vi "AdvancedConfig.vi"(8 "Error In":errorcluster, 11 "Config In":T1={"DAQ"={"Data"={"Live"={"t0"=timestamp(0 s since 1904-01-01), "dt"=1.0, "Y"=[]}, "Accumulated"={"t0"=timestamp(0 s since 1904-01-01), "dt"=1.0, "Y"=[]}, "Averaged"={"t0"=timestamp(0 s since 1904-01-01), "dt"=1.0, "Y"=[]}, "data array"=[], "live time array"=[], "Live (decimated)"={"t0"=timestamp(0 s since 1904-01-01), "dt"=1.0, "Y"=[]}}, "Config"={"Input Config"=0, "Card"=enum."USB-6211", "100% Reflectance Standard (V)"=0.0, "Input Channel"="Dev1/ai0", "Average number of points"=0.0, "Trigger Level (V)"=0.0, "Rate (Hz)"=0, "End Time (s)"=0.0}, "Indicators"={"Final number of points"=0.0, "Number of samples"=0.0, "dt"=0.0, "Shots"=0, "Shot counter"=0, "Test counter"=0, "Background level (V)"=0.0, "DAQ task"="", "timestamp of data"=timestamp(0 s since 1904-01-01), "Test Type"=enum."A-Test"}}, "Shutter"={"Open command string"="", "VISA"={"Timeout (ms)"=0, "Resource Name"="", "Baud Rate"=0, "Data Bits"=0, "Parity"=0, "Stop Bits"=0, "Flow Control"=0}}, "Monochromator"={"Type"=enum."Oriel", "Wavelength (nm)"=0.0, "Grating, gr/mm"=enum."2400", "Grating mode"=enum."Unknown", "Spectrum mode"={"Spectrum mode?"=FALSE, "Start wavelength (nm)"=0.0, "End wavelength (nm)"=0.0, "Wavelength step (nm)"=0.0, "Wavelength array"=[], "array index"=0}, "PTI"={"Delay before read (ms)"=0, "Mono 1"={"Timeout (ms)"=0, "Resource Name"="", "Baud Rate"=0, "Data Bits"=0, "Parity"=0, "Stop Bits"=0, "Flow Control"=0}, "Mono 2"={"Timeout (ms)"=0, "Resource Name"="", "Baud Rate"=0, "Data Bits"=0, "Parity"=0, "Stop Bits"=0, "Flow Control"=0}, "Two PTI Monochromators?"=FALSE}, "Oriel (custom)"={"reference"=refnum}, "Force wavelength confirmation (PTI)?"=FALSE}, "Test"={"Config"={"Amplification Factor"=0.0, "100% Reflectance Standard"=0.0, "Calculation Method"=enum."Reflectance", "Option to discard new data?"=FALSE, "Mode"=enum."Spectrum", "Number of Averages"=0, "B Test?"=FALSE}, "Indicators"={"DAQ Background Level (V)"=0.0, "A-Test Counter"=0, "B-Test Counter"=0, "Type"=enum."A-Test", "Scope Background Level (Amps)"=2.0, "TAS only?"=FALSE}}, "Scope"={"Config"={"VISA Resource"="", "Model"=enum."DPO 3012", "Timebase"=0.0, "Timeout (ms)"=0, "TAS"={"Vertical Range (V)"=0.0, "Vertical Offset (0.0 divs)"=0.0, "Bandwidth"=0, "Probe Attenuation (10.0)"=0.0, "Vertical Coupling"=0, "Impedance"=0, "Multiplication factor"=0.0, "Channel"=enum."Channel 1"}, "TPC"={"Vertical Range (V)"=0.0, "Vertical Offset (0.0 divs)"=0.0, "Bandwidth"=0, "Probe Attenuation (10.0)"=0.0, "Vertical Coupling"=0, "Impedance"=0, "Multiplication factor"=0.0, "Channel"=enum."Channel 1"}, "Trigger"={"Mode"=enum."Laser (TAS)", "Source "=enum."Channel 1", "PIA"={"Test LEDs"=FALSE, "LED line"="", "LED off (s)"=0.0, "LED on (s)"=0.0}, "Threshold (V)"=0.0}}, "Indicators"={"Setup"={"Final number of points"=0.0, "Pretrigger points"=0.0, "Number of readouts"=0, "Model"={"Acquisition Type"=0, "Record length (points)"=0, "Averages on scope"=0, "Average number of points"=0.0}}, "Timestamp of Data"=timestamp(0 s since 1904-01-01)}, "Data"={"TPC"={"Live data"={"t0"=timestamp(0 s since 1904-01-01), "dt"=1.0, "Y"=[]}, "Averaged data"={"t0"=timestamp(0 s since 1904-01-01), "dt"=1.0, "Y"=[]}, "Accumulated data"={"t0"=timestamp(0 s since 1904-01-01), "dt"=1.0, "Y"=[]}, "Final data"={"t0"=timestamp(0 s since 1904-01-01), "dt"=1.0, "Y"=[]}}, "TAS"={"Live data"={"t0"=timestamp(0 s since 1904-01-01), "dt"=1.0, "Y"=[]}, "Averaged data"={"t0"=timestamp(0 s since 1904-01-01), "dt"=1.0, "Y"=[]}, "Accumulated data"={"t0"=timestamp(0 s since 1904-01-01), "dt"=1.0, "Y"=[]}, "Final data"={"t0"=timestamp(0 s since 1904-01-01), "dt"=1.0, "Y"=[]}}, "Time arrays"={"Time array (decimated)"=[], "waveform"={"t0"=timestamp(0 s since 1904-01-01), "dt"=1.0, "Y"=[]}}}, "Test"={"Config"={"Amplification Factor"=2.0, "100% Reflectance Standard"=2.0, "Calculation Method"=enum."Reflectance", "Option to discard new data?"=FALSE, "Mode"=enum."Spectrum", "Number of Averages"=0, "B Test?"=FALSE}, "Indicators"={"DAQ Background Level (V)"=2.0, "A-Test Counter"=2, "B-Test Counter"=2, "Type"=enum."A-Test", "Scope Background Level (Amps)"=2.0, "TAS only?"=FALSE}}}, "Colour wheel"={"Reference"=0, "Colour Wheel Wavelengths"=[], "Waveform Index"=0, "COM Port"="", "Enabled?"=FALSE}, "File IO"={"Output Folder"=path "", "Error file"=path "", "Config file"=path "", "File prefix"="", "Waveform read"={"t0"=timestamp(0 s since 1904-01-01), "dt"=1.0, "Y"=[]}}} {"Scope"."Test"."Config"."Number of Averages" min=0; "Scope"."Indicators"."Setup"."Model"."Record length (points)" items=["1000"=1, "10,000"=10, "100,000"=100, "1,000,000"=1000, "5,000,000"=5000, "10,000,000"=10000]; "Scope"."Indicators"."Setup"."Model"."Acquisition Type" items=["Sample", "Peak Detect", "Hi Res", "Envelope", "Average"]; "Scope"."Config"."Trigger"."Threshold (V)" format="%#_3f"; "Scope"."Config"."TPC"."Impedance" items=["1M", "75", "50"]; "Scope"."Config"."TPC"."Vertical Coupling" items=["AC", "DC", "Ground"]; "Scope"."Config"."TPC"."Bandwidth" items=["FULL", "250 MHz", "150 MHz", "20 MHz"]; "Scope"."Config"."TAS"."Impedance" items=["1M", "75", "50"]; "Scope"."Config"."TAS"."Vertical Coupling" items=["AC", "DC", "Ground"]; "Scope"."Config"."TAS"."Bandwidth" items=["FULL", "250 MHz", "150 MHz", "20 MHz"]; "Scope"."Config"."Timebase" format="%^#_3e"; "Test"."Config"."Number of Averages" min=0; "Monochromator"."PTI"."Mono 2"."Flow Control" items=["1.0"=10, "1.5"=15, "2.0"=20]; "Monochromator"."PTI"."Mono 2"."Stop Bits" items=["None", "Odd", "Even", "Mark", "Space"]; "Monochromator"."PTI"."Mono 2"."Parity" items=["None", "Odd", "Even", "Mark", "Space"]; "Monochromator"."PTI"."Mono 1"."Flow Control" items=["1.0"=10, "1.5"=15, "2.0"=20]; "Monochromator"."PTI"."Mono 1"."Stop Bits" items=["None", "Odd", "Even", "Mark", "Space"]; "Monochromator"."PTI"."Mono 1"."Parity" items=["None", "Odd", "Even", "Mark", "Space"]; "Shutter"."VISA"."Flow Control" items=["None"=0, "XON/XOFF"=1, "RTS/CTS"=2, "DTR/DSR"=4]; "Shutter"."VISA"."Stop Bits" items=["1.0"=10, "1.5"=15, "2.0"=20]; "Shutter"."VISA"."Parity" items=["None", "Odd", "Even", "Mark", "Space"]; "DAQ"."Config"."Input Config" items=["default"=-1, "RSE"=10083, "NRSE"=10078, "Differential"=10106, "Pseudodifferential"=12529]}) -> (0 "Error Out":errorcluster)   [LabVIEW 2017, in "UI.lvlib"]
uses:
  UI.lvlib
  Controls/Move shutter button.ctl
  System Control/CTLs/Params.ctl
  DAQ/Controls/Params.ctl
  DAQ/Controls/DAQ Config.ctl
  DAQ/Controls/DAQ Indicators.ctl
  System Control/CTLs/Test Type.ctl
  Shutter Module/Controls/Params.ctl
  Monochromator/Controls/VISA parameters.ctl
  Monochromator/Controls/Params.ctl
  Monochromator/Controls/Type.ctl
  Monochromator/Controls/GratingValues.ctl
  Monochromator/Controls/Grating.ctl
  Monochromator/PTI/Controls/Params.ctl
  Monochromator/Custom Oriel drivers/Controls/Params.ctl
  C:/Optical Software Code V1.6.1.1/Optical Software Code/Modules/Monochromator/Cornerstone.dll
  Monochromator/Cornerstone.dll
  System Control/CTLs/Test params.ctl
  System Control/CTLs/Test Controls.ctl
  System Control/CTLs/Test indicators.ctl
  Scope/Controls/Params.ctl
  Scope/Controls/Models.ctl
  Scope/Controls/TPC.ctl
  Scope/Controls/Channels.ctl
  Trigger/Controls/Params.ctl
  Trigger/Controls/Mode.ctl
  Trigger/Controls/Trigger channels.ctl
  Scope/Controls/Acquisition type.ctl
  Scope/Controls/Record length.ctl
  Scope/Controls/Data.ctl
  Scope/Controls/Channel data.ctl
  Colour Wheel/Controls/Params.ctl
  File IO/Controls/Params.ctl
  Controls/Config Command [enum].ctl
  File IO/Controls/Config Cluster.ctl
  Shutter Module/Shutter.lvlib
  File IO/File IO.lvlib
  <vilib>/Utility/config.llb/NI_LVConfig.lvlib
  Colour Wheel/Colour Wheel.lvlib
  System Control/Main controller.lvlib
  Trigger/Trigger.lvlib
  Scope/Scope.lvlib
  Monochromator/Custom Oriel drivers/Oriel (custom drivers).lvlib
  Serial comms/Serial comms.lvlib
  Monochromator/PTI/PTI.lvlib
  Monochromator/Monochromator.lvlib
  DAQ/DAQ.lvlib
panel:
  out "Current Config:":path
  in  "Load Config Button":bool
  in  "Save Config Button":bool
  in  "Exit Button":bool
  in  "Tab Control":T30(tab)=enum."Colour Wheel"
  in  "Error Log File":path
  out "Pretrigger points":dbl
  out "Final number of points":dbl
  in  "Scope.Config":T31 {"Trigger"."Threshold (V)" format="%#_3f"; "TPC"."Impedance" items=["1M", "75", "50"]; "TPC"."Vertical Coupling" items=["AC", "DC", "Ground"]; "TPC"."Bandwidth" items=["FULL", "250 MHz", "150 MHz", "20 MHz"]; "TAS"."Impedance" items=["1M", "75", "50"]; "TAS"."Vertical Coupling" items=["AC", "DC", "Ground"]; "TAS"."Bandwidth" items=["FULL", "250 MHz", "150 MHz", "20 MHz"]}
  in  "Scope Model Settings":T32 {"Record length (points)" items=["1000"=1, "10,000"=10, "100,000"=100, "1,000,000"=1000, "5,000,000"=5000, "10,000,000"=10000]; "Acquisition Type" items=["Sample", "Peak Detect", "Hi Res", "Envelope", "Average"]}
  in  "DAQ Controls":T3={"Input Config"=10106, "Card"=enum."USB-6251", "100% Reflectance Standard (V)"=1.0, "Input Channel"="Dev1/ai0", "Average number of points"=10.0, "Trigger Level (V)"=0.2, "Rate (Hz)"=1250000, "End Time (s)"=10.0} {"Input Config" items=["default"=-1, "RSE"=10083, "NRSE"=10078, "Differential"=10106, "Pseudodifferential"=12529]}
  out "DAQ Indicators":T4={"Final number of points"=100.0, "Number of samples"=10000.0, "dt"=5e-06, "Shots"=10, "Shot counter"=10, "Test counter"=10, "Background level (V)"=0.0, "DAQ task"="", "timestamp of data"=timestamp(0 s since 1904-01-01), "Test Type"=enum."A-Test"}
  in  "Desired Wavelength:":dbl min=0.0 max=1600.0 step=1.0
  in  "Move Monochromator Button":bool
  in  "Monochromator Type":T9=enum."PTI"
  in  "Wavelength (nm)":dbl
  in  "Grating, gr/mm":T10
  in  "Monochromator Grating mode":T11=enum."IR"
  in  "PTI":T12={"Delay before read (ms)"=50, "Mono 1"={"Timeout (ms)"=1000, "Resource Name"="COM1", "Baud Rate"=9600, "Data Bits"=8, "Parity"=0, "Stop Bits"=10, "Flow Control"=0}, "Mono 2"={"Timeout (ms)"=1000, "Resource Name"="COM1", "Baud Rate"=9600, "Data Bits"=8, "Parity"=0, "Stop Bits"=10, "Flow Control"=0}, "Two PTI Monochromators?"=FALSE} {"Mono 2"."Flow Control" items=["None"=0, "XON/XOFF"=1, "RTS/CTS"=2, "DTR/DSR"=4]; "Mono 2"."Stop Bits" items=["1.0"=10, "1.5"=15, "2.0"=20]; "Mono 2"."Parity" items=["None", "Odd", "Even", "Mark", "Space"]; "Mono 1"."Flow Control" items=["None"=0, "XON/XOFF"=1, "RTS/CTS"=2, "DTR/DSR"=4]; "Mono 1"."Stop Bits" items=["1.0"=10, "1.5"=15, "2.0"=20]; "Mono 1"."Parity" items=["None", "Odd", "Even", "Mark", "Space"]}
  in  "Waveform Index":i32
  in  "Colour Wheel Settings":T28={"Reference"=0, "Colour Wheel Wavelengths"=[], "Waveform Index"=0, "COM Port"="COM1", "Enabled?"=FALSE}
  in  "Move Colour Wheel Button":T33
  in  "Shutter Settings":cluster{"Open command string":string, "VISA":T7}={"Open command string"="+100\\s10\\n", "VISA"={"Timeout (ms)"=1000, "Resource Name"="", "Baud Rate"=9600, "Data Bits"=9600, "Parity"=8, "Stop Bits"=0, "Flow Control"=10}} {"VISA"."Flow Control" items=["None"=0, "XON/XOFF"=1, "RTS/CTS"=2, "DTR/DSR"=4]; "VISA"."Stop Bits" items=["1.0"=10, "1.5"=15, "2.0"=20]; "VISA"."Parity" items=["None", "Odd", "Even", "Mark", "Space"]}
  in  "Move Shutter Button":T33
  # "Scope Settings"
  # "(Max = 250k/1.25M for\n6211/6251 DAQ cards)"
  # "Default is differential (connected ports are 15 and 16 on DAQ card).\n* For CH-TAS, input config should be RSE."
  # "Format: +100\\s20\\n OR \\F3\\002\\C1"
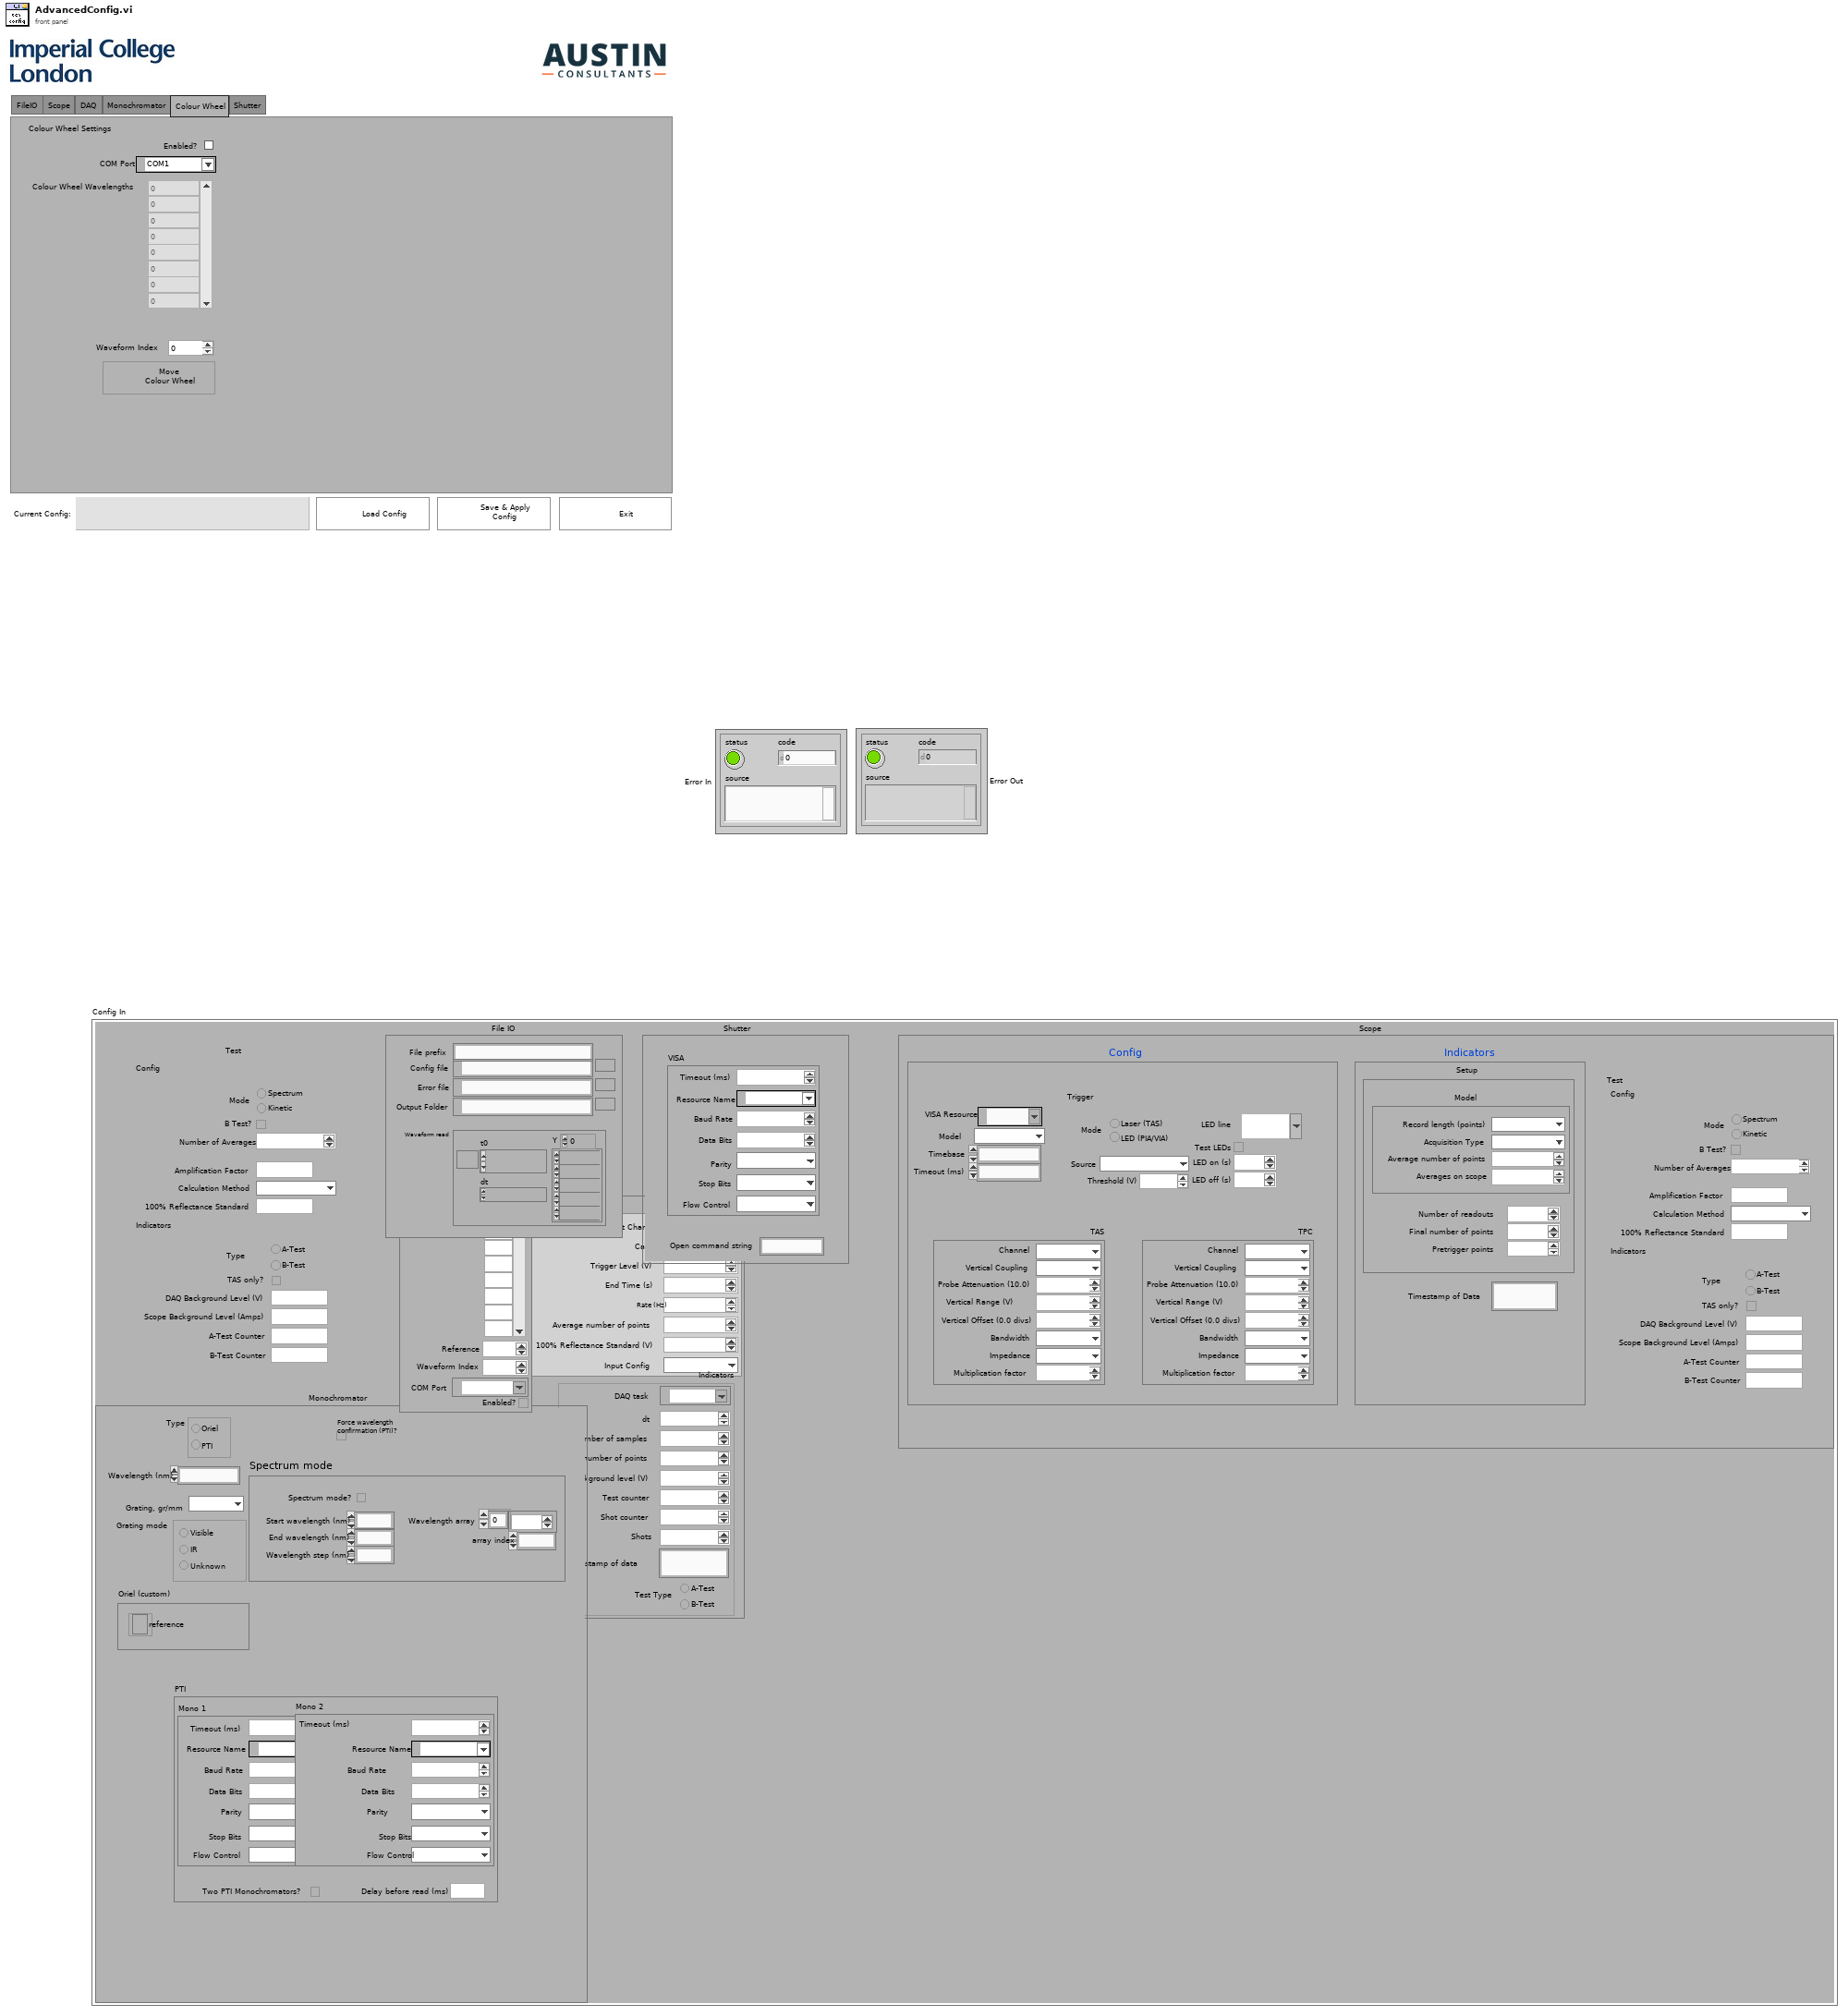
[diagram p1: front panel]
types:
  T1 = typedef "Main controller.lvlib/Params.ctl" = cluster{"DAQ":T2, "Shutter":T6, "Monochromator":T8, "Test":T14, "Scope":T17, "Colour wheel":T28, "File IO":T29}
  T2 = typedef "DAQ.lvlib/Params.ctl" = cluster{"Data":cluster{"Live":waveform(dbl), "Accumulated":waveform(dbl), "Averaged":waveform(dbl), "data array":dbl[], "live time array":dbl[], "Live (decimated)":waveform(dbl)}, "Config":T3, "Indicators":T4}
  T3 = typedef "DAQ.lvlib/DAQ Config.ctl" = cluster{"Input Config":i32, "Card":enum16{"USB-6211", "USB-6251", "USB-6361"}, "100% Reflectance Standard (V)":dbl, "Input Channel":tag, "Average number of points":dbl, "Trigger Level (V)":dbl, "Rate (Hz)":i32, "End Time (s)":dbl}
  T4 = typedef "DAQ.lvlib/DAQ Indicators.ctl" = cluster{"Final number of points":dbl, "Number of samples":dbl, "dt":dbl, "Shots":i32, "Shot counter":i32, "Test counter":i32, "Background level (V)":dbl, "DAQ task":refnum<k21>, "timestamp of data":timestamp, "Test Type":T5}
  T5 = typedef "Main controller.lvlib/Test Type.ctl" = enum32{"A-Test", "B-Test"}
  T6 = typedef "Shutter.lvlib/Params.ctl" = cluster{"Open command string":string, "VISA":T7}
  T7 = typedef "Serial comms.lvlib/VISA parameters.ctl" = cluster{"Timeout (ms)":u32, "Resource Name":refnum<visa-resource-name>, "Baud Rate":u32, "Data Bits":u16, "Parity":u16, "Stop Bits":u16, "Flow Control":u16}
  T8 = typedef "Monochromator.lvlib/Params.ctl" = cluster{"Type":T9, "Wavelength (nm)":dbl, "Grating, gr/mm":T10, "Grating mode":T11, "Spectrum mode":cluster{"Spectrum mode?":bool, "Start wavelength (nm)":dbl, "End wavelength (nm)":dbl, "Wavelength step (nm)":dbl, "Wavelength array":dbl[], "array index":u32}, "PTI":T12, "Oriel (custom)":T13, "Force wavelength confirmation (PTI)?":bool}
  T9 = typedef "Monochromator.lvlib/Type.ctl" = enum32{"Oriel", "PTI"}
  T10 = typedef "Monochromator.lvlib/GratingValues.ctl" = enum16{"2400", "1800", "1200", "600", "300", "150"}
  T11 = typedef "Monochromator.lvlib/Grating.ctl" = enum32{"Unknown", "Visible", "IR"}
  T12 = typedef "Monochromator.lvlib/PTI.lvlib/Params.ctl" = cluster{"Delay before read (ms)":u32, "Mono 1":T7, "Mono 2":T7, "Two PTI Monochromators?":bool}
  T13 = typedef "Monochromator.lvlib/Oriel (custom drivers).lvlib/Params.ctl" = cluster{"reference":refnum<k24>}
  T14 = typedef "Main controller.lvlib/Test params.ctl" = cluster{"Config":T15, "Indicators":T16}
  T15 = typedef "Main controller.lvlib/Test Controls.ctl" = cluster{"Amplification Factor":dbl, "100% Reflectance Standard":dbl, "Calculation Method":enum16{"Reflectance", "Transmission", "Kubelka-Munk"}, "Option to discard new data?":bool, "Mode":enum32{"Spectrum", "Kinetic"}, "Number of Averages":i32, "B Test?":bool}
  T16 = typedef "Main controller.lvlib/Test indicators.ctl" = cluster{"DAQ Background Level (V)":dbl, "A-Test Counter":i32, "B-Test Counter":i32, "Type":T5, "Scope Background Level (Amps)":dbl, "TAS only?":bool}
  T17 = typedef "Scope.lvlib/Params.ctl" = cluster{"Config":cluster{"VISA Resource":refnum<visa-resource-name>, "Model":T18, "Timebase":dbl, "Timeout (ms)":u32, "TAS":T19, "TPC":T19, "Trigger":T21}, "Indicators":cluster{"Setup":cluster{"Final number of points":dbl, "Pretrigger points":dbl, "Number of readouts":i32, "Model":cluster{"Acquisition Type":T24, "Record length (points)":T25, "Averages on scope":i32, "Average number of points":dbl}}, "Timestamp of Data":timestamp}, "Data":T26, "Test":T14}
  T18 = typedef "Scope.lvlib/Models.ctl" = enum16{"DPO 3012", "DPO 2012B", "TDS 3012C"}
  T19 = typedef "Scope.lvlib/TPC.ctl" = cluster{"Vertical Range (V)":dbl, "Vertical Offset (0.0 divs)":dbl, "Bandwidth":i32, "Probe Attenuation (10.0)":dbl, "Vertical Coupling":u16, "Impedance":u16, "Multiplication factor":dbl, "Channel":T20}
  T20 = typedef "Scope.lvlib/Channels.ctl" = enum16{"Channel 1", "Channel 2", "Channel 3", "Channel 4", "Math", "Reference A", "Reference B", "Reference C", "Reference D", "B1", "B2", "None"}
  T21 = typedef "Scope.lvlib/Trigger.lvlib/Params.ctl" = cluster{"Mode":T22, "Source ":T23, "PIA":cluster{"Test LEDs":bool, "LED line":tag, "LED off (s)":dbl, "LED on (s)":dbl}, "Threshold (V)":dbl}
  T22 = typedef "Scope.lvlib/Trigger.lvlib/Mode.ctl" = enum32{"Laser (TAS)", "LED (PIA/VIA)"}
  T23 = typedef "Scope.lvlib/Trigger.lvlib/Trigger channels.ctl" = enum16{"Channel 1", "Channel 2", "Channel 3", "Channel 4", "AC Line", "Aux", "Digital Channel 0", "Digital Channel 1", "Digital Channel 2", "Digital Channel 3", "Digital Channel 4", "Digital Channel 5", "Digital Channel 6", "Digital Channel 7", "Digital Channel 8", "Digital Channel 9", "Digital Channel 10", "Digital Channel 11", "Digital Channel 12", "Digital Channel 13", "Digital Channel 14", "Digital Channel 15", "RF"}
  T24 = typedef "Scope.lvlib/Acquisition type.ctl" = u16
  T25 = typedef "Scope.lvlib/Record length.ctl" = u32
  T26 = typedef "Scope.lvlib/Data.ctl" = cluster{"TPC":T27, "TAS":T27, "Time arrays":cluster{"Time array (decimated)":dbl[], "waveform":waveform(dbl)}}
  T27 = typedef "Scope.lvlib/Channel data.ctl" = cluster{"Live data":waveform(dbl), "Averaged data":waveform(dbl), "Accumulated data":waveform(dbl), "Final data":waveform(dbl)}
  T28 = typedef "Colour Wheel.lvlib/Params.ctl" = cluster{"Reference":i32, "Colour Wheel Wavelengths":dbl[], "Waveform Index":i32, "COM Port":refnum<visa-resource-name>, "Enabled?":bool}
  T29 = typedef "File IO.lvlib/Params.ctl" = cluster{"Output Folder":path, "Error file":path, "Config file":path, "File prefix":string, "Waveform read":waveform(dbl)}
  T30 = enum32{"FileIO", "Scope", "DAQ", "Monochromator", "Colour Wheel", "Shutter"}
  T31 = cluster{"VISA Resource":refnum<visa-resource-name>, "Model":T18, "Timebase":dbl, "Timeout (ms)":u32, "TAS":T19, "TPC":T19, "Trigger":T21}
  T32 = cluster{"Acquisition Type":T24, "Record length (points)":T25, "Averages on scope":i32, "Average number of points":dbl}
  T33 = typedef "UI.lvlib/Move shutter button.ctl" = bool
  T34 = typedef "UI.lvlib/Config Command [enum].ctl" = enum16{"Idle", "Update"}
  T35 = typedef "File IO.lvlib/Config Cluster.ctl" = cluster{"Test.Config":T15, "File IO":T29, "DAQ.Config":T3, "Monochromator":T8, "Scope.Config":cluster{"VISA Resource":refnum<visa-resource-name>, "Model":T18, "Timebase":dbl, "Timeout (ms)":u32, "TAS":T19, "TPC":T19, "Trigger":T21}, "Colour Wheel":T28, "Shutter":T6, "Scope.Setup.Model":cluster{"Acquisition Type":T24, "Record length (points)":T25, "Averages on scope":i32, "Average number of points":dbl}}
  T36 = typedef "NI_LVConfig.lvlib/Config Data RefNum.ctl" = refnum<k1>
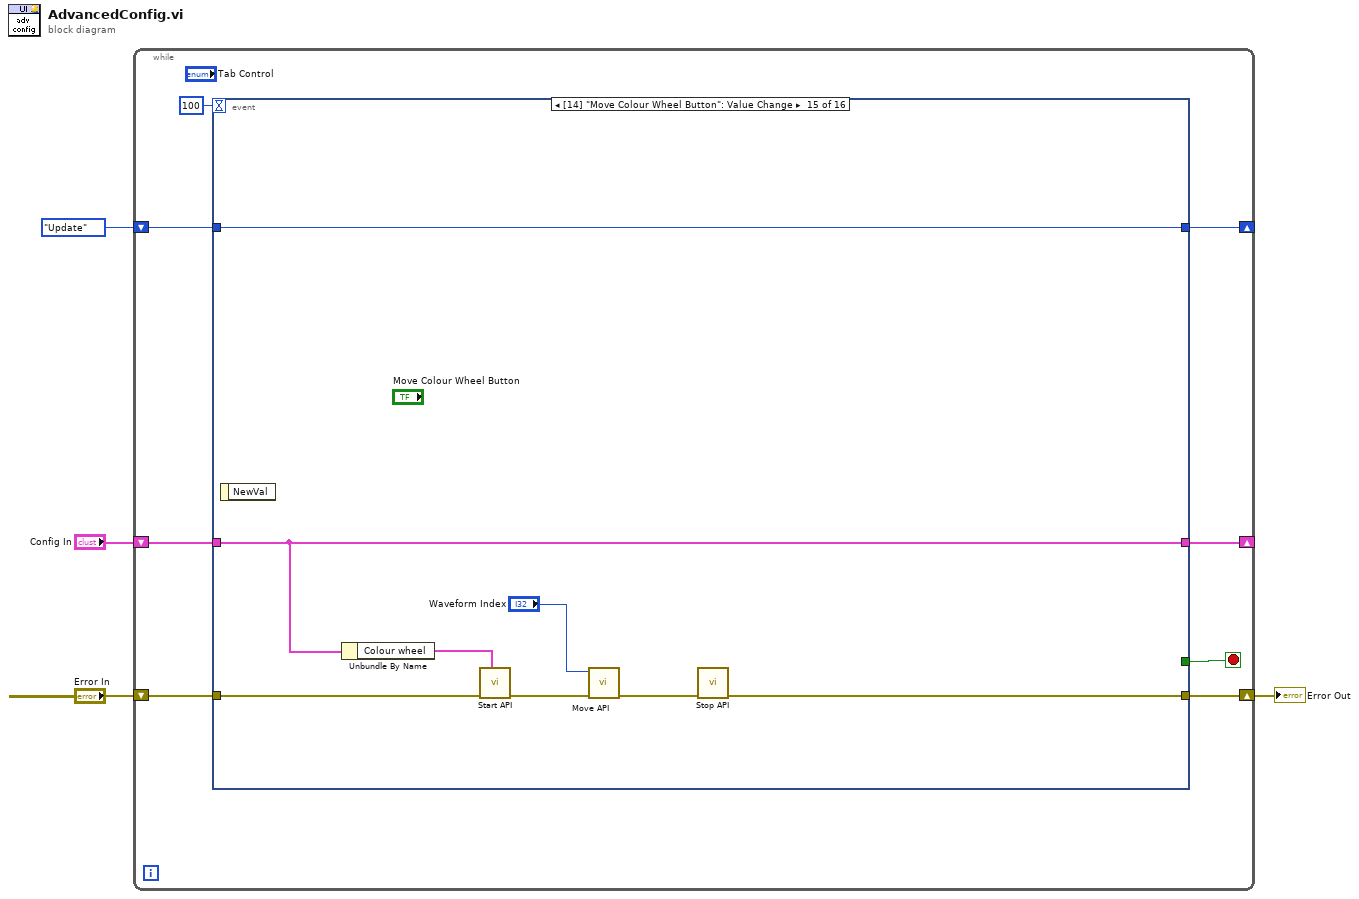
[diagram p0: block diagram]
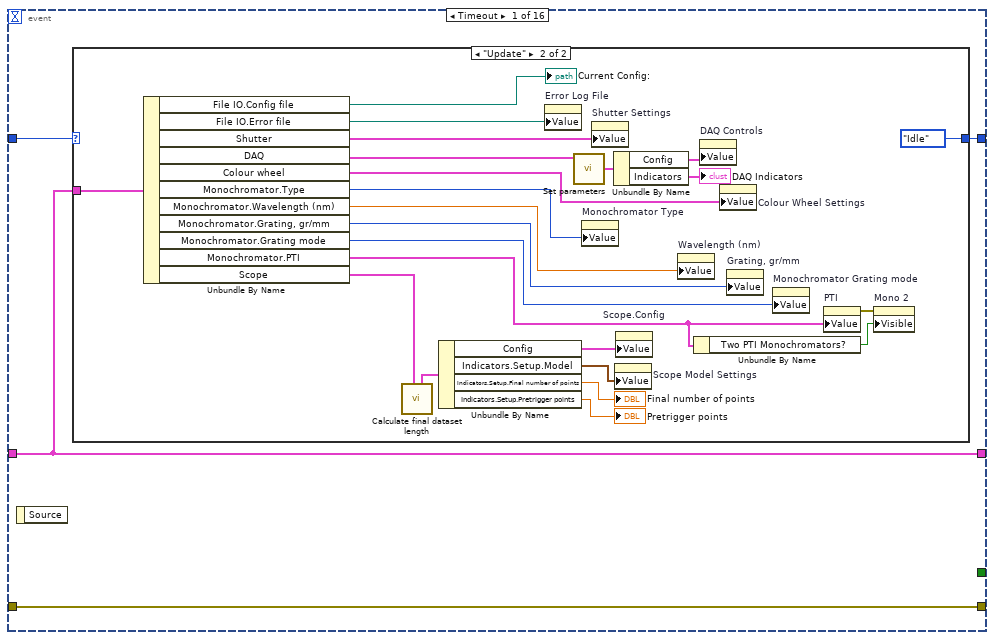
[diagram p2: hidden frame]
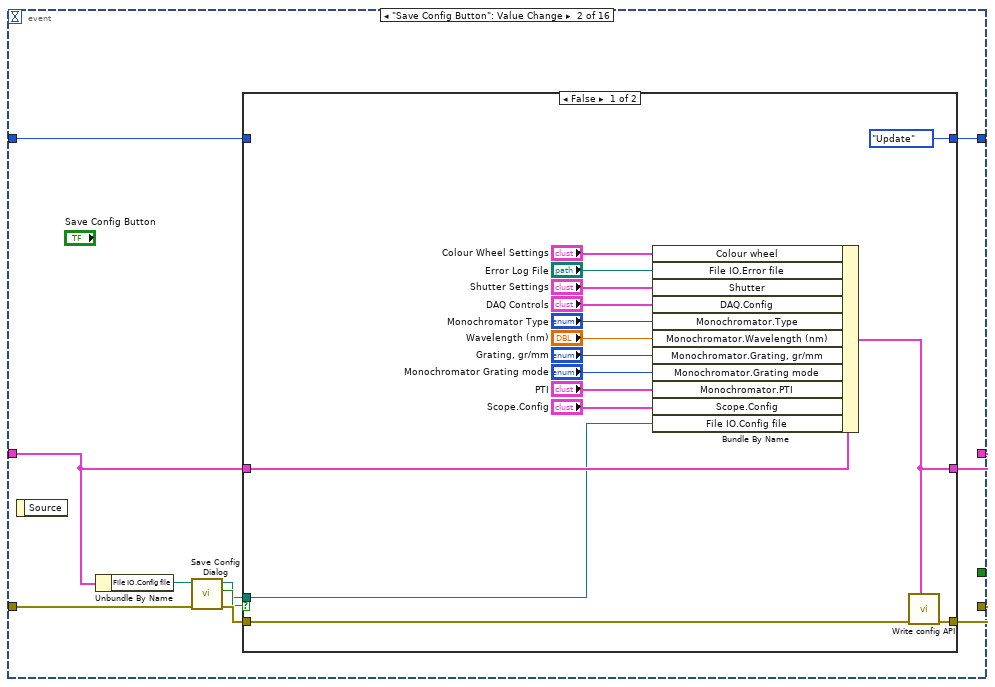
[diagram p4: hidden frame]
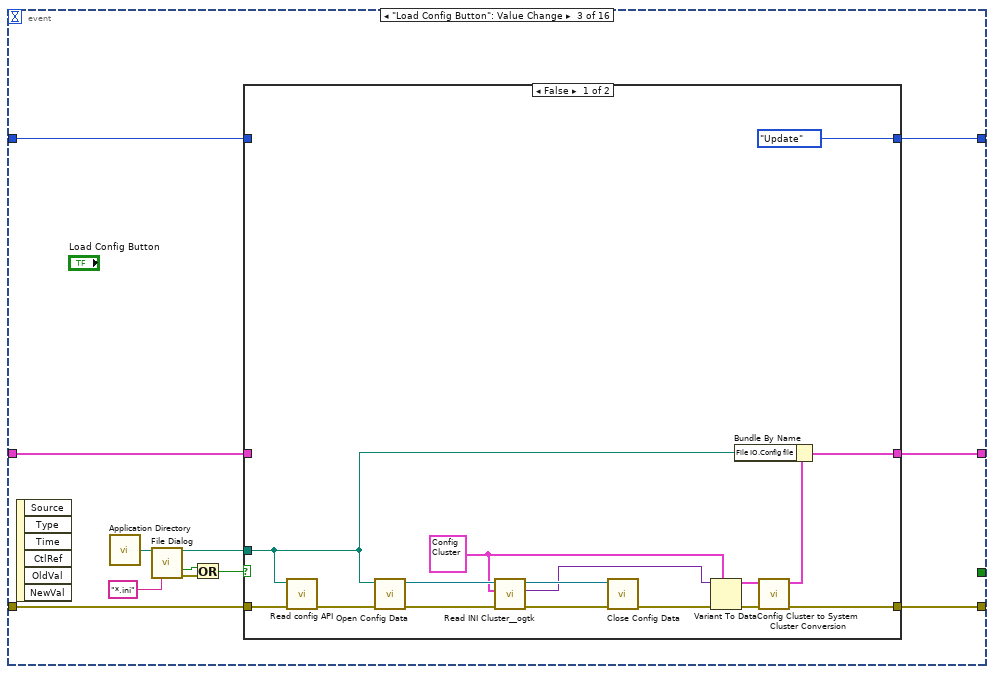
[diagram p6: hidden frame]
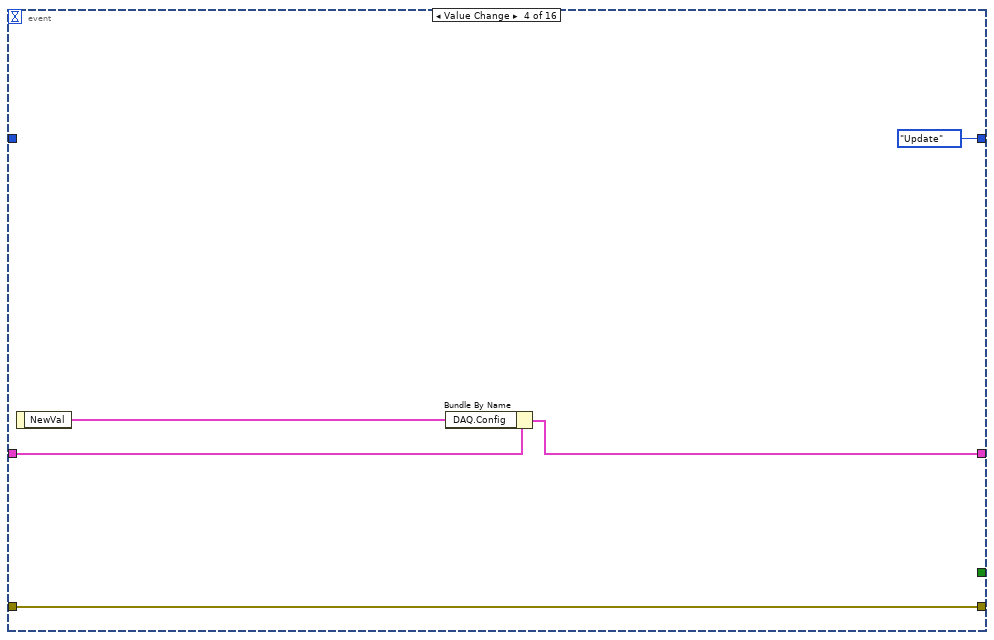
[diagram p8: hidden frame]
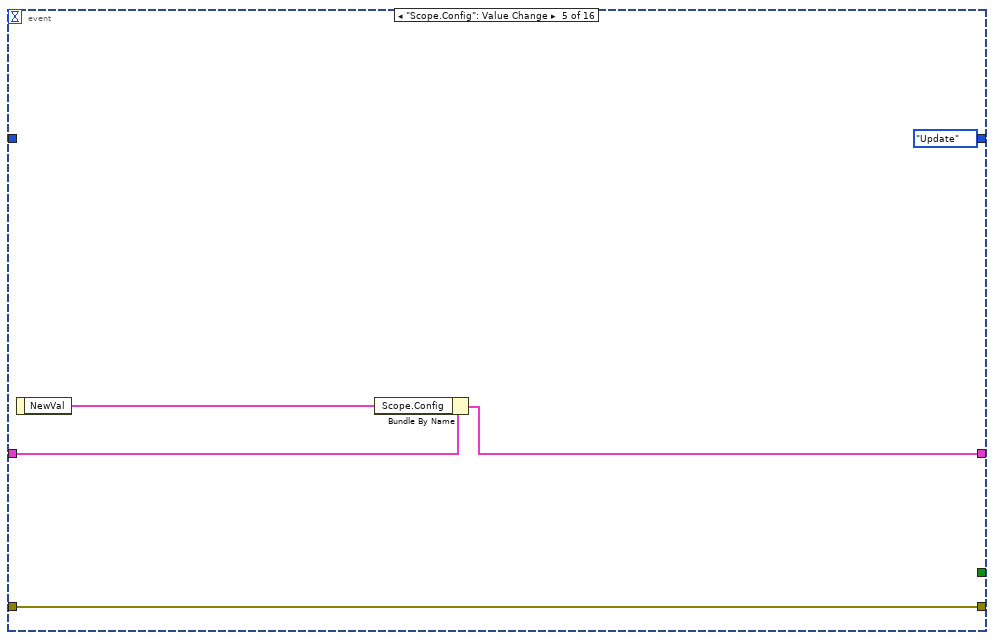
[diagram p9: hidden frame]
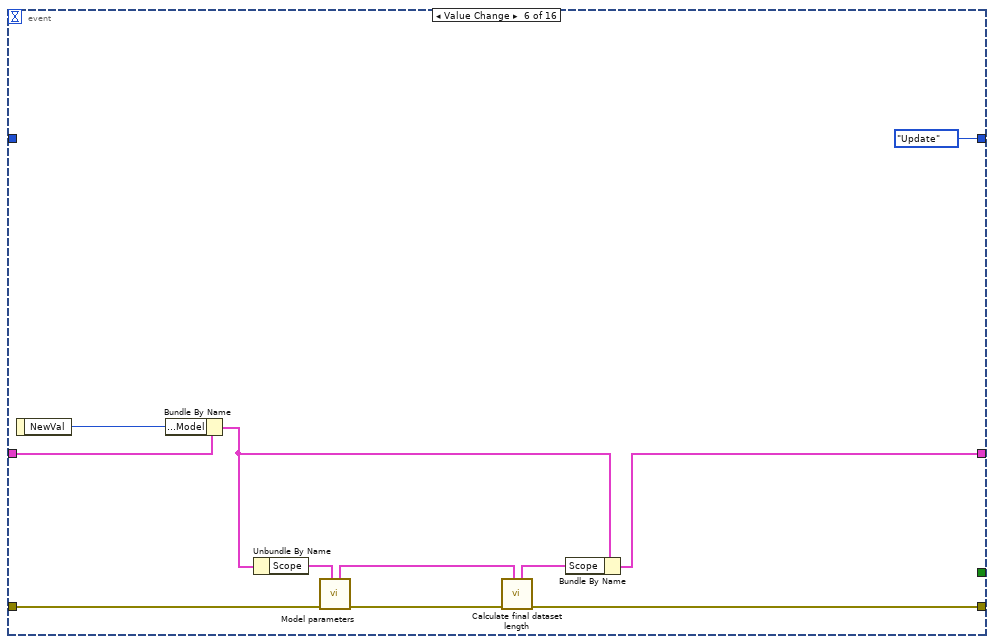
[diagram p10: hidden frame]
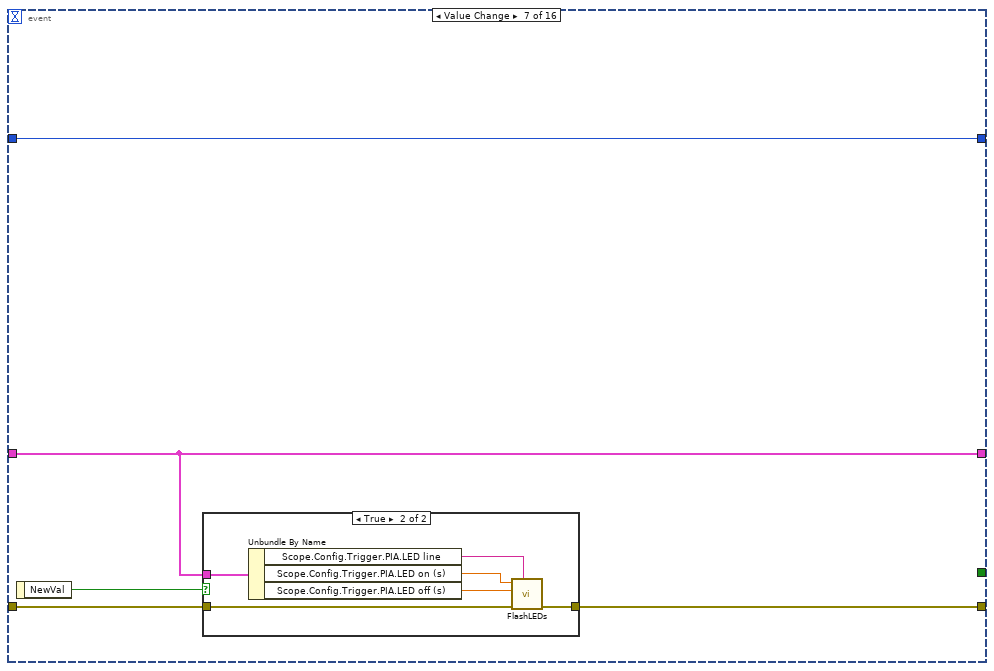
[diagram p11: hidden frame]
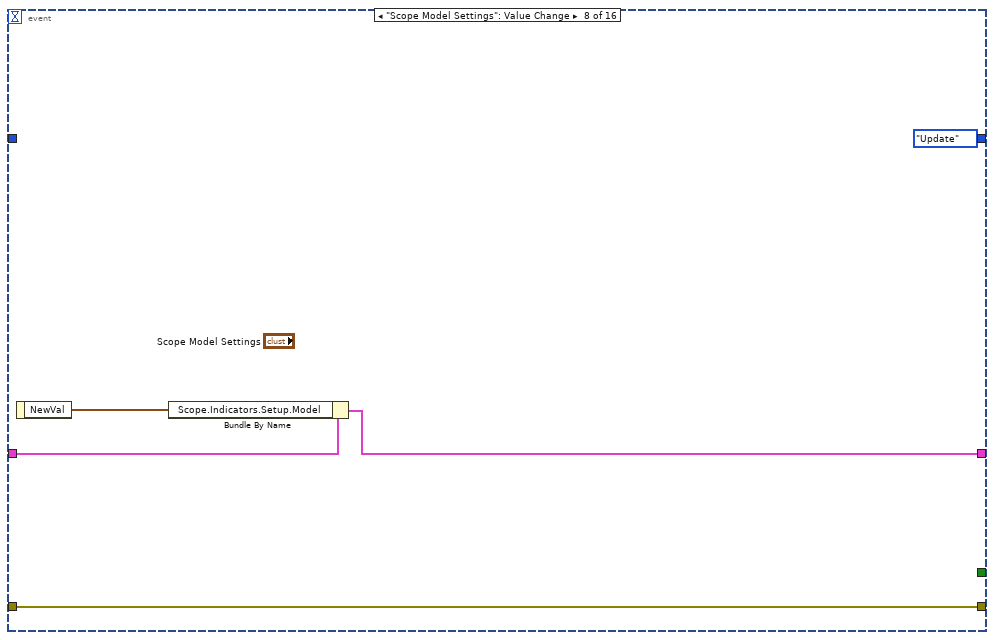
[diagram p13: hidden frame]
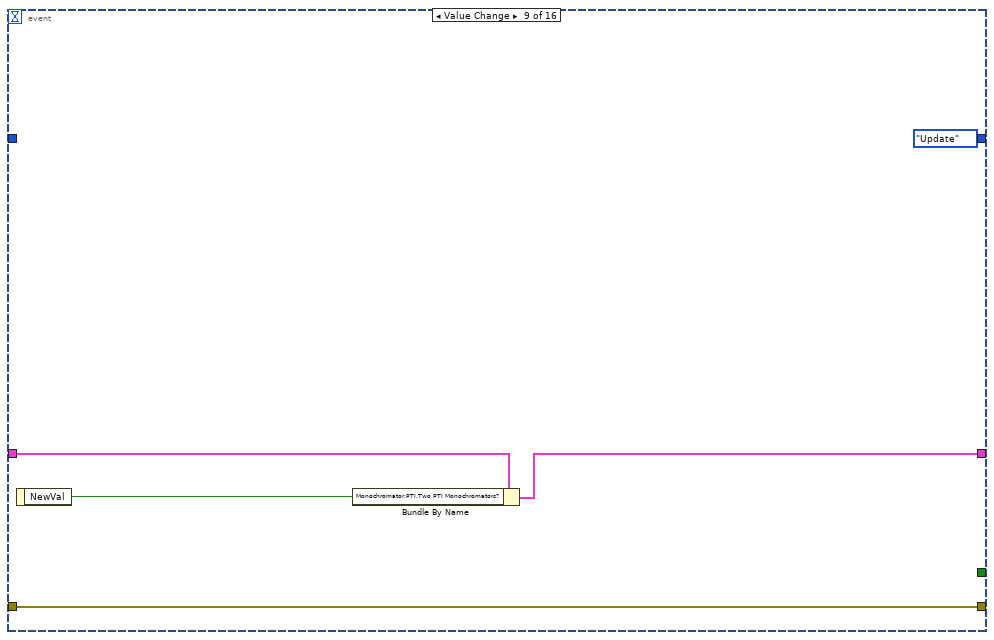
[diagram p14: hidden frame]
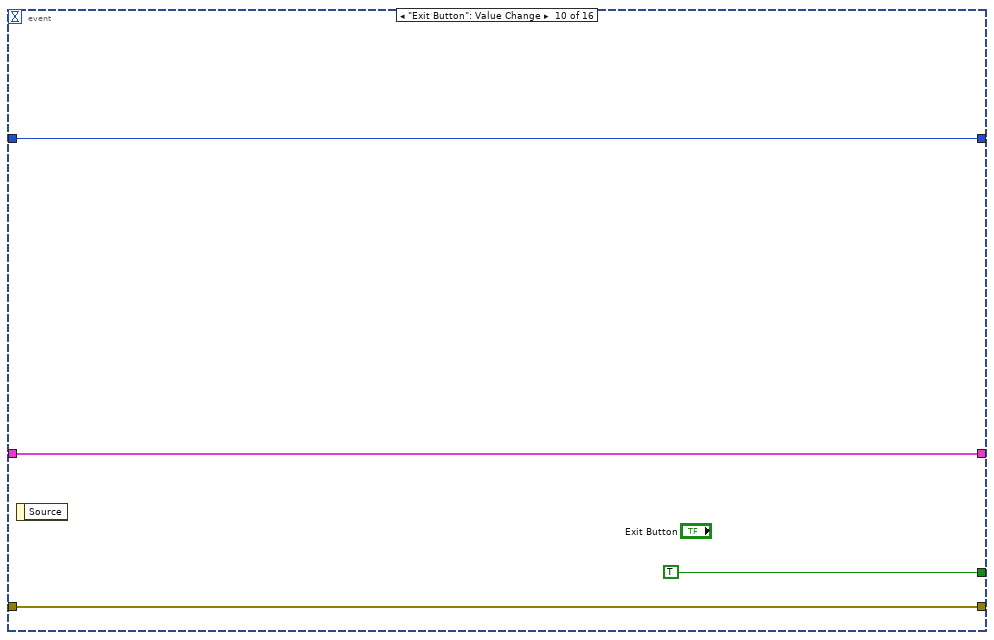
[diagram p15: hidden frame]
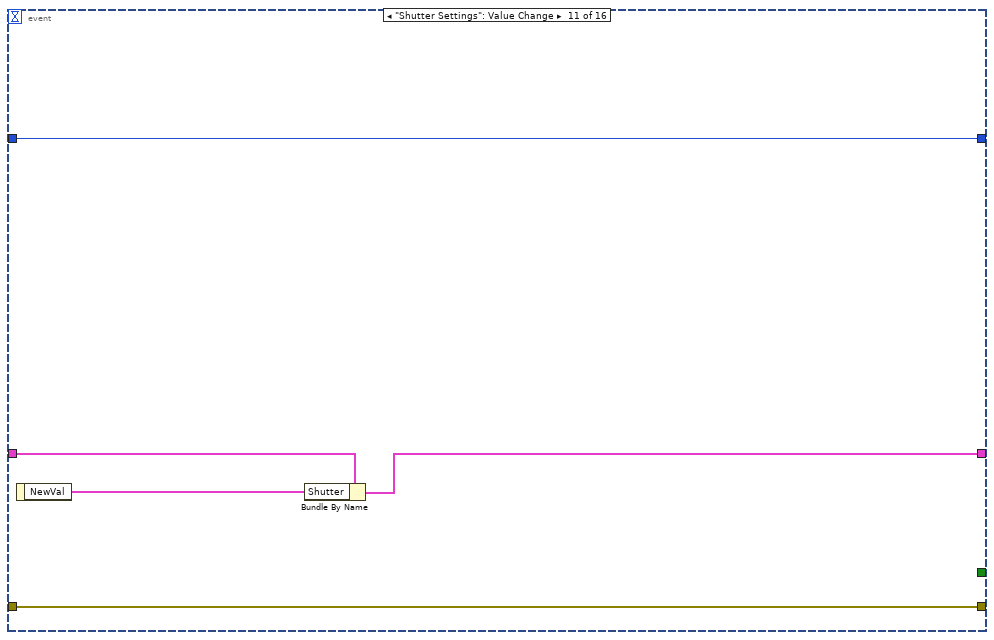
[diagram p16: hidden frame]
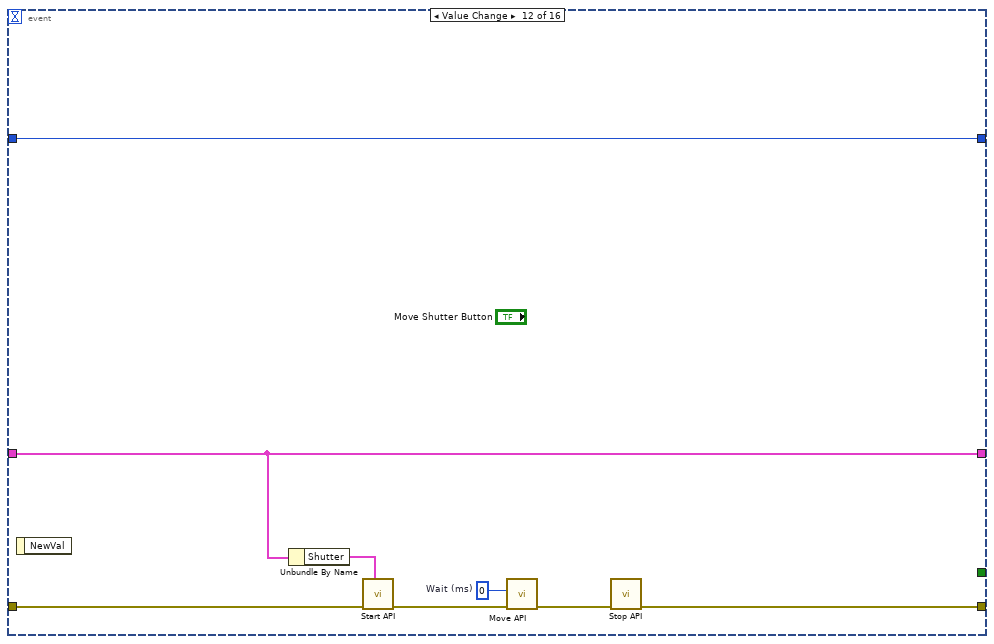
[diagram p17: hidden frame]
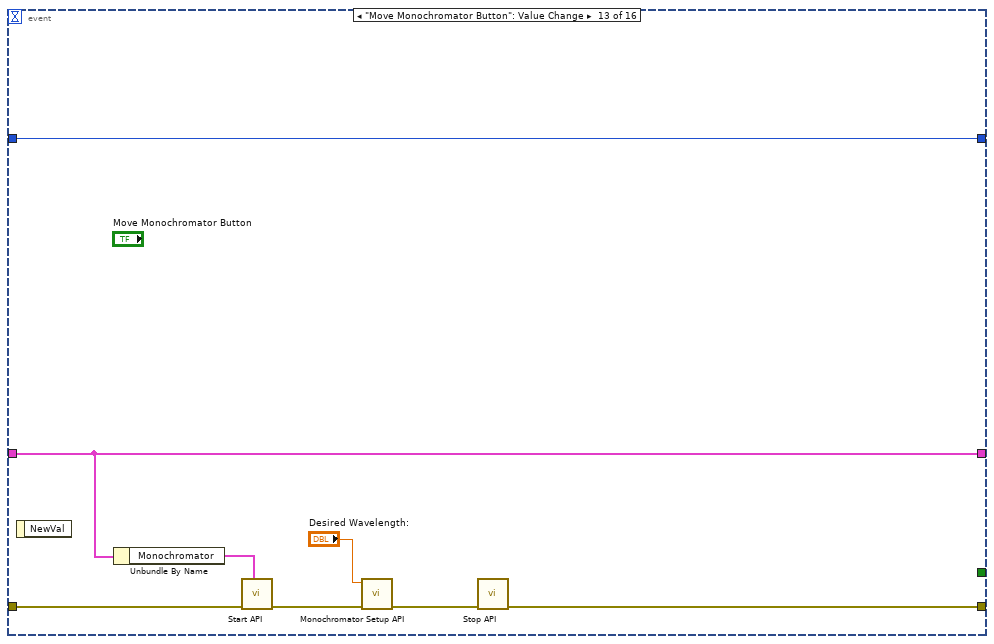
[diagram p18: hidden frame]
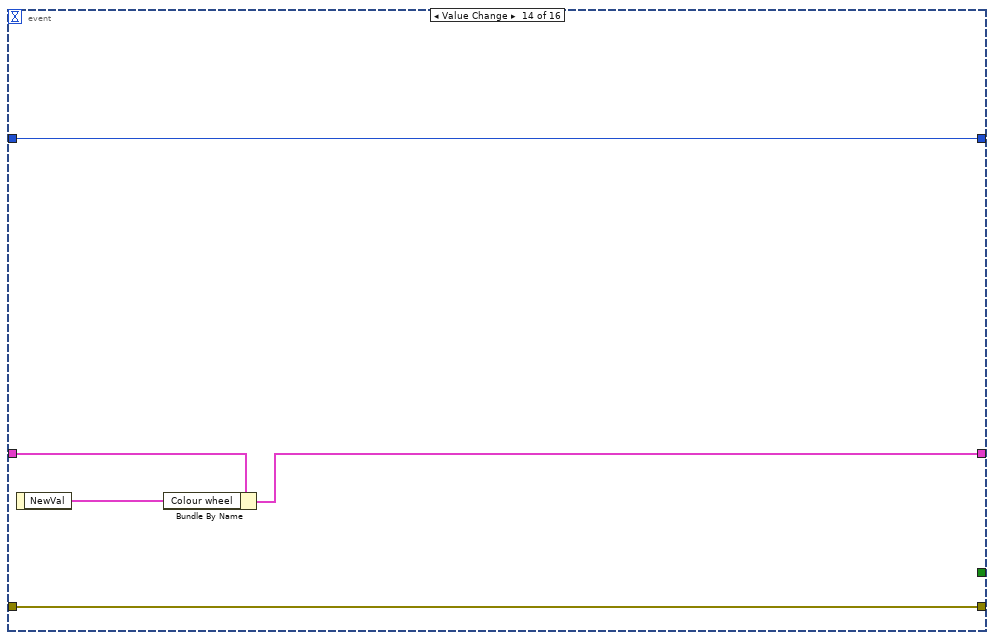
[diagram p19: hidden frame]
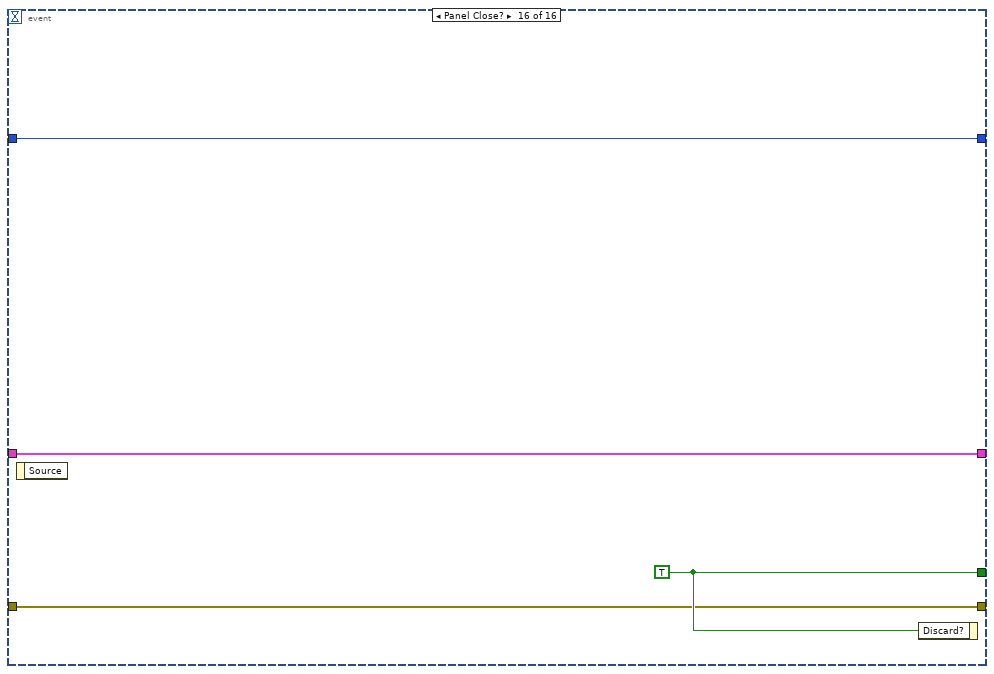
[diagram p20: hidden frame]
diagram:
  n1 = while {
    shift-right: [w12] -> w4
    shift-left: "Error In" -> [w8]
    shift-right: [w10] -> _
    shift-left: "Config In" -> [w9]
    shift-right: [w5] -> _
    shift-left: Config_Command_[enum]."Update" -> [w6]
    stop <- w11 stop-if-true
    n2 = event shown="[14] \"Move Colour Wheel Button\": Value Change" {
      selector: _ -> [_ _ _ _ _ _ _ _ _ _ _ _ _ _ _ _]
      dyn-events: _ -> [_ _ _ _ _ _ _ _ _ _ _ _ _ _ _ _]
      timeout: 100 -> [_ _ _ _ _ _ _ _ _ _ _ _ _ _ _ _]
      tunnel: [_ _ _ _ _ _ _ _ _ TRUE ("Discard?") _ _ _ _ _ w184] -> w11
      tunnel: [w16 w50 w78 w105 w110 w113 w124 w138 w143 w145 w152 w155 w164 w173 w176 w183] -> w12
      tunnel: w8 -> [w16 w48 w79 w105 w110 w120 w125 w138 w143 w145 w152 w156 w165 w173 w180 w183]
      tunnel: w9 -> [w15 w45 w72 w102 w109 w118 w122 w137 w142 w147 w150 w154 w163 w171 w178 w185]
      tunnel: [w15 w49 w73 w101 w108 w115 w122 w136 w141 w147 w149 w154 w163 w170 w178 w185] -> w10
      tunnel: w6 -> [w14 w42 w71 _ _ _ w126 _ _ w144 w148 w153 w168 w169 w181 w182]
      tunnel: [w13 w41 w70 Config_Command_[enum]."Update" Config_Command_[enum]."Update" Config_Command_[enum]."Update" w126 Config_Command_[enum]."Update" Config_Command_[enum]."Update" w144 w148 w153 w168 w169 w181 w182] -> w5
      event Timeout {
        n3 = event-data() -> ()  [unwired: 1 in, 1 out]
        n4 = case shown="\"Update\"" w14 {
          selector: w14 -> [w17 _]
          tunnel: w15 -> [_ w34]
          tunnel: [w17 Config_Command_[enum]."Idle"] -> w13
          frame "Idle", Default {
          }
          frame "Update" {
            n5 = Unbundle By Name(w34) -> ("File IO.Config file"=→"Current Config:":path, "File IO.Error file"=w35:path, "Shutter"=w36:T6, "DAQ"=w31:T2, "Colour wheel"=w23:T28, "Monochromator.Type"=w37:T9, "Monochromator.Wavelength (nm)"=w38:dbl, "Monochromator.Grating, gr/mm"=w39:T10, "Monochromator.Grating mode"=w40:T11, "Monochromator.PTI"=w26:T12, "Scope"=w19:T17)
            n6 = call "Calculate final dataset length.vi"("Scope in"=w19) -> ("Scope out"=w18:T17)  [unwired: 9 in, 1 out]
            n7 = Unbundle By Name(w18) -> ("Config"=w27:T31, "Indicators.Setup.Model"=w20:T32, "Indicators.Setup.Final number of points"=→"Final number of points":dbl, "Indicators.Setup.Pretrigger points"=→"Pretrigger points":dbl)
            n8 = property on="Error Log File" class="Path"("Value"=w35) -> ()  [unwired: 2 in, 2 out]
            n9 = call "Set parameters.vi"("DAQ"=w31) -> ("DAQ out"=w30:T2)  [unwired: 9 in, 1 out]
            n10 = property on="Monochromator Type" class="RadioBtnsControl (strict)"("Value"=w37) -> ()  [unwired: 2 in, 2 out]
            n11 = property on="Shutter Settings" class="Clust (strict)"("Value"=w36) -> ()  [unwired: 2 in, 2 out]
            n12 = Unbundle By Name(w30) -> ("Config"=w29:T3, "Indicators"=→"DAQ Indicators":T4)
            n13 = property on="Scope Model Settings" class="Clust (strict)"("Value"=w20) -> ()  [unwired: 2 in, 2 out]
            n14 = property on="Scope.Config" class="Clust (strict)"("Value"=w27) -> ()  [unwired: 2 in, 2 out]
            n15 = property on="Wavelength (nm)" class="DigNum (strict)"("Value"=w38) -> ()  [unwired: 2 in, 2 out]
            n16 = Unbundle By Name(w26) -> ("Two PTI Monochromators?"=w24:bool)
            n17 = property on="DAQ Controls" class="Clust (strict)"("Value"=w29) -> ()  [unwired: 2 in, 2 out]
            n18 = property on="Colour Wheel Settings" class="Clust (strict)"("Value"=w23) -> ()  [unwired: 2 in, 2 out]
            n19 = property on="Grating, gr/mm" class="Enum (strict)"("Value"=w39) -> ()  [unwired: 2 in, 2 out]
            n20 = property on="Monochromator Grating mode" class="RadioBtnsControl (strict)"("Value"=w40) -> ()  [unwired: 2 in, 2 out]
            n21 = property on="PTI" class="Clust (strict)"("Value"=w26) -> (error out=w25:errorcluster)  [unwired: 2 in, 1 out]
            n22 = property on="Mono 2" class="Clust (strict)"(error in=w25, "Visible"=w24) -> ()  [unwired: 1 in, 2 out]
          }
        }
      }
      event "Save Config Button": Value Change {
        n23 = event-data() -> ()  [unwired: 1 in, 1 out]
        n24 = Unbundle By Name(w45) -> ("File IO.Config file"=w44:path)
        n25 = call "Save Config Dialog.vi"("error in (no error)"=w48, "Current Config Path"=w44) -> ("error out"=w47:errorcluster, "Cancelled"=w46:bool, "New Config Path"=w43:path)  [unwired: 7 in]
        n26 = case shown="False" w46 {
          tunnel: w47 -> [w66 w68]
          tunnel: [w65 w68] -> w50
          tunnel: w45 -> [w63 w69]
          tunnel: [w56 w69] -> w49
          tunnel: w43 -> [w53 _]
          tunnel: w42 -> [_ w67]
          tunnel: [Config_Command_[enum]."Update" w67] -> w41
          frame False {
            n27 = Bundle By Name(cluster=w63, "Colour wheel"="Colour Wheel Settings", "File IO.Error file"="Error Log File", "Shutter"="Shutter Settings", "DAQ.Config"="DAQ Controls", "Monochromator.Type"="Monochromator Type", "Monochromator.Wavelength (nm)"="Wavelength (nm)", "Monochromator.Grating, gr/mm"="Grating, gr/mm", "Monochromator.Grating mode"="Monochromator Grating mode", "Monochromator.PTI"="PTI", "Scope.Config"="Scope.Config", "File IO.Config file"=w53) -> (w56:T1)
            n28 = call "Write config API.vi"("System parameters"=w56, "Error In"=w66) -> ("Error Out"=w65:errorcluster)  [unwired: 9 in]
          }
          frame True {
          }
        }
      }
      event "Load Config Button": Value Change {
        n29 = event-data() -> ()  [unwired: 1 in, 6 out]
        n30 = call <vilib>:"Application Directory.vi"() -> ("Application Directory"=w81:path)
        n31 = call "File Dialog"("start path"=w81, "pattern (all files)"="*.ini" ("pattern label")) -> ("selected path"=w77:path, "cancelled"=w75:bool, "error out"=w76:errorcluster)  [unwired: 10 in, 1 out]
        n32 = Or(x=w75, y=w76) -> (x .or. y?=w74:bool)
        n33 = case shown="False" w74 {
          tunnel: w79 -> [w97 w100]
          tunnel: [w83 w100] -> w78
          tunnel: w77 -> [w84 _]
          tunnel: [w82 w99] -> w73
          tunnel: w72 -> [_ w99]
          tunnel: w71 -> [_ w98]
          tunnel: [Config_Command_[enum]."Update" w98] -> w70
          frame False {
            w86 = T35 {"Test.Config"={"Amplification Factor"=0.0, "100% Reflectance Standard"=0.0, "Calculation Method"=enum."Reflectance", "Option to discard new data?"=FALSE, "Mode"=enum."Kinetic", "Number of Averages"=0, "B Test?"=FALSE}, "File IO"={"Output Folder"=path "C:/Users/Abigail/Documents/Imperial Optical software/Optical Software Code Simplified/Output", "Error file"=path "Error Log.txt", "Config file"=path "Config.ini", "File prefix"="", "Waveform read"={"t0"=timestamp(0 s since 1904-01-01), "dt"=1.0, "Y"=[]}}, "DAQ.Config"={"Input Config"=10106, "Card"=enum."USB-6251", "100% Reflectance Standard (V)"=1.0, "Input Channel"="Dev1/ai0", "Average number of points"=10.0, "Trigger Level (V)"=0.2, "Rate (Hz)"=1250000, "End Time (s)"=10.0}, "Monochromator"={"Type"=enum."PTI", "Wavelength (nm)"=600.0, "Grating, gr/mm"=enum."1200", "Grating mode"=enum."Unknown", "Spectrum mode"={"Spectrum mode?"=FALSE, "Start wavelength (nm)"=0.0, "End wavelength (nm)"=0.0, "Wavelength step (nm)"=0.0, "Wavelength array"=[], "array index"=0}, "PTI"={"Delay before read (ms)"=50, "Mono 1"={"Timeout (ms)"=1000, "Resource Name"="COM1", "Baud Rate"=9600, "Data Bits"=8, "Parity"=0, "Stop Bits"=10, "Flow Control"=0}, "Mono 2"={"Timeout (ms)"=1000, "Resource Name"="COM1", "Baud Rate"=9600, "Data Bits"=8, "Parity"=0, "Stop Bits"=10, "Flow Control"=0}, "Two PTI Monochromators?"=FALSE}, "Oriel (custom)"={"reference"=refnum}, "Force wavelength confirmation (PTI)?"=FALSE}, "Scope.Config"={"VISA Resource"="", "Model"=enum."DPO 3012", "Timebase"=0.0, "Timeout (ms)"=0, "TAS"={"Vertical Range (V)"=0.0, "Vertical Offset (0.0 divs)"=0.0, "Bandwidth"=0, "Probe Attenuation (10.0)"=0.0, "Vertical Coupling"=0, "Impedance"=0, "Multiplication factor"=0.0, "Channel"=enum."Channel 1"}, "TPC"={"Vertical Range (V)"=0.0, "Vertical Offset (0.0 divs)"=0.0, "Bandwidth"=0, "Probe Attenuation (10.0)"=0.0, "Vertical Coupling"=0, "Impedance"=0, "Multiplication factor"=0.0, "Channel"=enum."Channel 1"}, "Trigger"={"Mode"=enum."Laser (TAS)", "Source "=enum."Channel 1", "PIA"={"Test LEDs"=FALSE, "LED line"="", "LED off (s)"=0.0, "LED on (s)"=0.0}, "Threshold (V)"=0.0}}, "Colour Wheel"={"Reference"=0, "Colour Wheel Wavelengths"=[], "Waveform Index"=0, "COM Port"="", "Enabled?"=FALSE}, "Shutter"={"Open command string"="+100\\s10\\n", "VISA"={"Timeout (ms)"=1000, "Resource Name"="", "Baud Rate"=9600, "Data Bits"=9600, "Parity"=8, "Stop Bits"=0, "Flow Control"=10}}, "Scope.Setup.Model"={"Acquisition Type"=0, "Record length (points)"=0, "Averages on scope"=0, "Average number of points"=0.0}} ("Config Cluster")
            n34 = call "Read config API.vi"("Error In"=w97, "Config file"=w84) -> ("Error Out"=w85:errorcluster)  [unwired: 9 in]
            n35 = call <vilib>:"Open Config Data.vi"("error in (no error)"=w85, "configuration file path"=w84) -> ("error out"=w94:errorcluster, "refnum"=w95:T36)  [unwired: 7 in, 1 out]
            n36 = call <userlib>:"Read INI Cluster__ogtk.vi"("error in (no error)"=w94, "INI Fomatted Cluster Type"=w86, "refnum"=w95) -> ("error out"=w93:errorcluster, "INI Fomatted Cluster"=w91:variant, "dup refnum"=w92:T36)  [unwired: 4 in, 2 out]
            n37 = call <vilib>:"Close Config Data.vi"("error in (no error)"=w93, "refnum"=w92) -> ("error out"=w90:errorcluster)  [unwired: 8 in, 1 out]
            n38 = Variant To Data(error in=w90, type=w86, Variant=w91) -> (data=w89:T35, error out=w87:errorcluster)
            n39 = call "Config Cluster to System Cluster Conversion.vi"("error in (no error)"=w87, "Config Cluster"=w89) -> ("error out"=w83:errorcluster, "System Cluster"=w88:T1)  [unwired: 8 in]
            n40 = Bundle By Name(cluster=w88, "File IO.Config file"=w84) -> (w82:T1)
          }
          frame True {
          }
        }
      }
      event Value Change {
        n41 = event-data() -> ("NewVal"=w104:T3)  [unwired: 1 in]
        n42 = Bundle By Name(cluster=w102, "DAQ.Config"=w104) -> (w101:T1)
      }
      event "Scope.Config": Value Change {
        n43 = event-data() -> ("NewVal"=w107:T31)  [unwired: 1 in]
        n44 = Bundle By Name(cluster=w109, "Scope.Config"=w107) -> (w108:T1)
      }
      event Value Change {
        n45 = event-data() -> ("NewVal"=w117:T18)  [unwired: 1 in]
        n46 = Bundle By Name(cluster=w118, "Scope.Config.Model"=w117) -> (w116:T1)
        n47 = Unbundle By Name(w116) -> ("Scope"=w119:T17)
        n48 = call "Model parameters.vi"("Scope"=w119, "error in"=w120) -> ("error out"=w114:errorcluster, "Scope out"=w112:T17)  [unwired: 8 in]
        n49 = call "Calculate final dataset length.vi"("Scope in"=w112, "error in (no error)"=w114) -> ("error out"=w113:errorcluster, "Scope out"=w111:T17)  [unwired: 8 in]
        n50 = Bundle By Name(cluster=w116, "Scope"=w111) -> (w115:T1)
      }
      event Value Change {
        n51 = event-data() -> ("NewVal"=w123:bool)  [unwired: 1 in]
        n52 = case shown="True" w123 {
          tunnel: w125 -> [w127 w133]
          tunnel: [w127 w132] -> w124
          tunnel: w122 -> [_ w131]
          frame False {
          }
          frame True {
            n53 = Unbundle By Name(w131) -> ("Scope.Config.Trigger.PIA.LED line"=w130:tag, "Scope.Config.Trigger.PIA.LED on (s)"=w129:dbl, "Scope.Config.Trigger.PIA.LED off (s)"=w128:dbl)
            n54 = call "FlashLEDs.vi"("LED line"=w130, "error in (no error)"=w133, "LED off (s)"=w128, "LED on (s)"=w129) -> ("error out"=w132:errorcluster)  [unwired: 7 in]
          }
        }
      }
      event "Scope Model Settings": Value Change {
        n55 = event-data() -> ("NewVal"=w135:T32)  [unwired: 1 in]
        n56 = Bundle By Name(cluster=w137, "Scope.Indicators.Setup.Model"=w135) -> (w136:T1)
      }
      event Value Change {
        n57 = event-data() -> ("NewVal"=w140:bool)  [unwired: 1 in]
        n58 = Bundle By Name(cluster=w142, "Monochromator.PTI.Two PTI Monochromators?"=w140) -> (w141:T1)
      }
      event "Exit Button": Value Change {
        n59 = event-data() -> ()  [unwired: 1 in, 1 out]
      }
      event "Shutter Settings": Value Change {
        n60 = event-data() -> ("NewVal"=w151:cluster{"Open command string":string, "VISA":T7})  [unwired: 1 in]
        n61 = Bundle By Name(cluster=w150, "Shutter"=w151) -> (w149:T1)
      }
      event Value Change {
        w157 = u32 0  # Wait (ms)
        n62 = event-data() -> ()  [unwired: 1 in, 1 out]
        n63 = Unbundle By Name(w154) -> ("Shutter"=w159:T6)
        n64 = call "Start API.vi"("Shutter"=w159, "Error In"=w156) -> ("Error Out"=w158:errorcluster)  [unwired: 9 in]
        n65 = call "Move API.vi"("Error In"=w158, "Wait (ms)"=w157) -> ("Error Out"=w160:errorcluster)  [unwired: 9 in]
        n66 = call "Stop API.vi"("Error In"=w160) -> ("Error Out"=w155:errorcluster)  [unwired: 10 in]
      }
      event "Move Monochromator Button": Value Change {
        n67 = event-data() -> ()  [unwired: 1 in, 1 out]
        n68 = Unbundle By Name(w163) -> ("Monochromator"=w162:T8)
        n69 = call "Start API.vi"("Monochromator"=w162, "Error In"=w165) -> ("Error Out"=w167:errorcluster)  [unwired: 9 in]
        n70 = call "Monochromator Setup API.vi"("Error In"=w167, "wavelength"="Desired Wavelength:") -> ("Error Out"=w166:errorcluster)  [unwired: 9 in]
        n71 = call "Stop API.vi"("Error In"=w166) -> ("Error Out"=w164:errorcluster)  [unwired: 10 in]
      }
      event Value Change {
        n72 = event-data() -> ("NewVal"=w172:T28)  [unwired: 1 in]
        n73 = Bundle By Name(cluster=w171, "Colour wheel"=w172) -> (w170:T1)
      }
      event Value Change {
        n74 = event-data() -> ()  [unwired: 1 in, 1 out]
        n75 = Unbundle By Name(w178) -> ("Colour wheel"=w179:T28)
        n76 = call "Start API.vi"("Colour wheel"=w179, "Error In"=w180) -> ("Error Out"=w175:errorcluster)  [unwired: 9 in]
        n77 = call "Move API.vi"("Error In"=w175, "Index"="Waveform Index") -> ("Error Out"=w177:errorcluster)  [unwired: 9 in]
        n78 = call "Stop API.vi"("Error In"=w177) -> ("Error Out"=w176:errorcluster)  [unwired: 10 in]
      }
      event Panel Close? {
        w184 = TRUE
        n79 = event-data() -> ()  [unwired: 1 in, 1 out]
        n80 = event-data("Discard?"=w184) -> ()  [unwired: 1 in, 1 out]
      }
    }
  }
  "Error Out" <- w4
